vi "Check Serial Read --Unit Test.vi"(11 "Read buffer In":string) -> (3 "Results out":cluster{"message":string, "Passed?":bool})   [LabVIEW 2021]
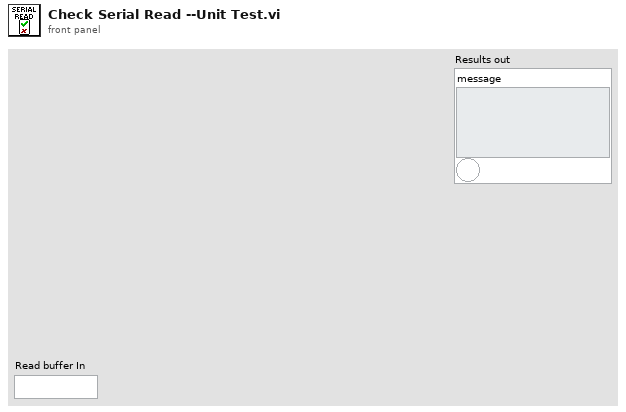
[diagram p1: front panel]
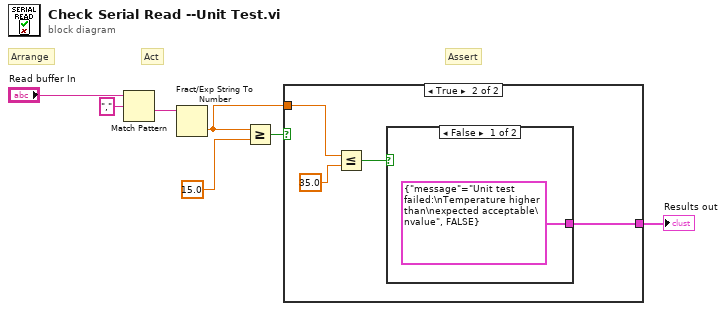
[diagram p0: block diagram]
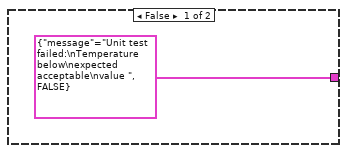
[diagram p2: hidden frame]
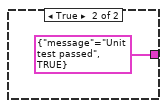
[diagram p3: hidden frame]
diagram:
  # "Assert"
  # "Act"
  # "Arrange"
  n1 = Match Pattern(string="Read buffer In", regular expression=",") -> (after substring=w5:string)  [unwired: 1 in, 3 out]
  n2 = Fract/Exp String To Number(string=w5) -> (number=w2:dbl)  [unwired: 3 in, 1 out]
  n3 = Greater Or Equal?(x=w2, y=15.0) -> (x >= y?=w3:bool)
  n4 = case shown="True" w3 {
    tunnel: w2 -> [_ w12]
    tunnel: [cluster{"message":string, bool} {"message"="Unit test failed:\nTemperature below\nexpected acceptable\nvalue ", FALSE} w9] -> w1
    frame False {
    }
    frame True {
      n5 = Less Or Equal?(x=w12, y=35.0) -> (x <= y?=w10:bool)
      n6 = case shown="False" w10 {
        tunnel: [cluster{"message":string, bool} {"message"="Unit test failed:\nTemperature higher than\nexpected acceptable\nvalue", FALSE} cluster{"message":string, bool} {"message"="Unit test passed", TRUE}] -> w9
        frame False {
        }
        frame True {
        }
      }
    }
  }
  "Results out" <- w1
